vi "Config Comparator Normal.vi"(0 "VISA resource name":refnum<visa-resource-name>, 1 "Element (1: Element 1)":u16(ring)=1 items=["", "Element1", "Element2", "Element3", "Sigma"], 5 "Channel (1)":u16=1 min=1 max=4 step=1, 7 "Normal Limit Item (1: V)":u16(ring)=1 items=["OFF", "V", "A", "W", "VA", "var", "PF", "Phase", "VHz", "AHz", "Wh", "Wh+", "Wh-", "Ah", "Ah+", "Ah-", "Math", "Vpk", "Apk"], 9 "Normal Limit Value (0)":dbl min=-9999000000.0 max=9999000000.0 format="%^.3e", 11 "error in (no error)":errorcluster) -> (4 "VISA resource name out":refnum<visa-resource-name>, 15 "error out":errorcluster)   [LabVIEW 2013, in "Yokogawa WT200 Series.lvlib"]
doc: "This VI sends the comparator limit values commands of normal measurement to the WT200 Series.\n\nNote : It needs /CMP option."
uses:
  <instrlib>/Yokogawa WT200 Series/Yokogawa WT200 Series.lvlib
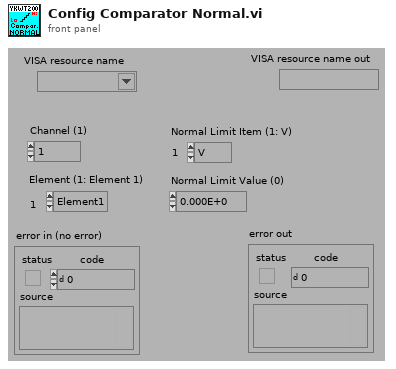
[diagram p1: front panel]
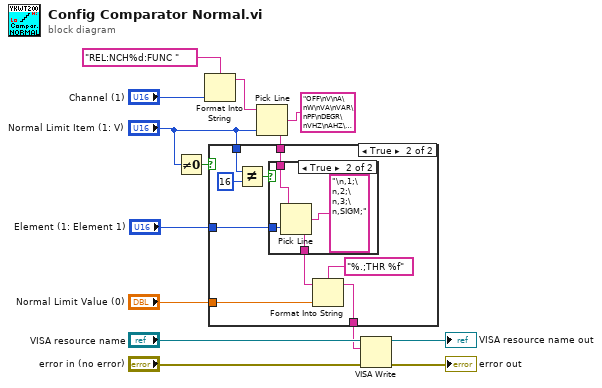
[diagram p0: block diagram]
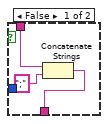
[diagram p3: hidden frame]
diagram:
  n1 = Not Equal To 0?(x="Normal Limit Item (1: V)") -> (x != 0?=w2:bool)
  n2 = Format Into String(format string="REL:NCH%d:FUNC ", "Channel (1)") -> (resulting string=w5:string)  [unwired: 2 in, 1 out]
  n3 = Pick Line(string ("")=w5, multi-line string="OFF\nV\nA\nW\nVA\nVAR\nPF\nDEGR\nVHZ\nAHZ\nWH\nWHP\nWHM\nAH\nAHP\nAHM\nMATH\nVPK\nAPK", line index="Normal Limit Item (1: V)") -> (output string=w6:string)
  n4 = case shown="True" w2 {
    tunnel: [w15 w24] -> w4
    tunnel: "Normal Limit Item (1: V)" -> [_ w22]
    tunnel: w6 -> [w15 w19]
    tunnel: "Normal Limit Value (0)" -> [_ w17]
    tunnel: "Element (1: Element 1)" -> [_ w16]
    frame False {
      # "OFF"
    }
    frame True {
      n5 = Not Equal?(x=w22, y=u16 16) -> (x != y?=w23:bool)
      n6 = case shown="True" w23 {
        tunnel: w19 -> [w26 w30]
        tunnel: [w25 w29] -> w20
        tunnel: w16 -> [_ w28]
        frame False {
          n7 = Concatenate Strings(w26, ";") -> (w25:string)
        }
        frame True {
          n8 = Pick Line(string ("")=w30, multi-line string="\n,1;\n,2;\n,3;\n,SIGM;" ("ÏÙÁ×²Ý•¶Žš—ñ"), line index=w28) -> (output string=w29:string)
        }
      }
      n9 = Format Into String(format string="%.;THR %f", initial string=w20, w17) -> (resulting string=w24:string)  [unwired: 1 in, 1 out]
    }
  }
  n10 = VISA Write(VISA resource name="VISA resource name", write buffer=w4, error in (no error)="error in (no error)") -> (VISA resource name out=→"VISA resource name out":refnum<visa-resource-name>, error out=→"error out":errorcluster)  [unwired: 1 out]
